vi "SetAOrange.vi"(8 "error in (no error)":errorcluster, 10 "output range":cluster{"output high":dbl, "output low":dbl}={"output high"=nan, "output low"=0.0}, 11 "MotorCtrl in":refnum<class "MotorControl.lvclass">) -> (0 "error out":errorcluster, 2 "output range dup":cluster{"output high":dbl, "output low":dbl}, 3 "MotorCtrl out":refnum<class "MotorControl.lvclass">)   [LabVIEW 2015, in "MotorControl.lvclass"]
uses:
  MotorControl.lvclass
  MotorControl.lvclass/MotorControl.ctl
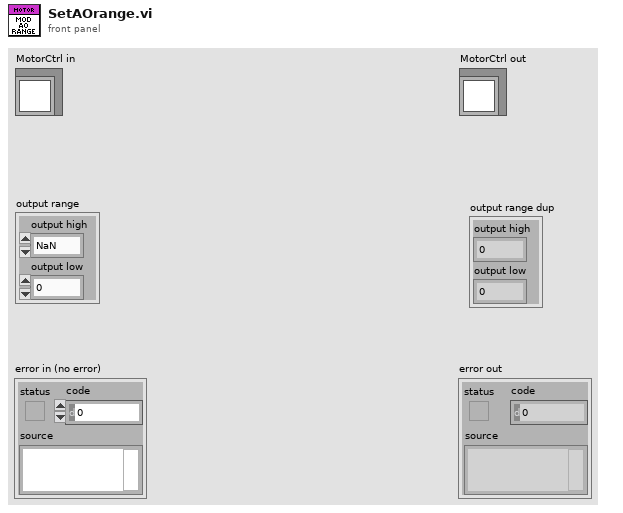
[diagram p1: front panel]
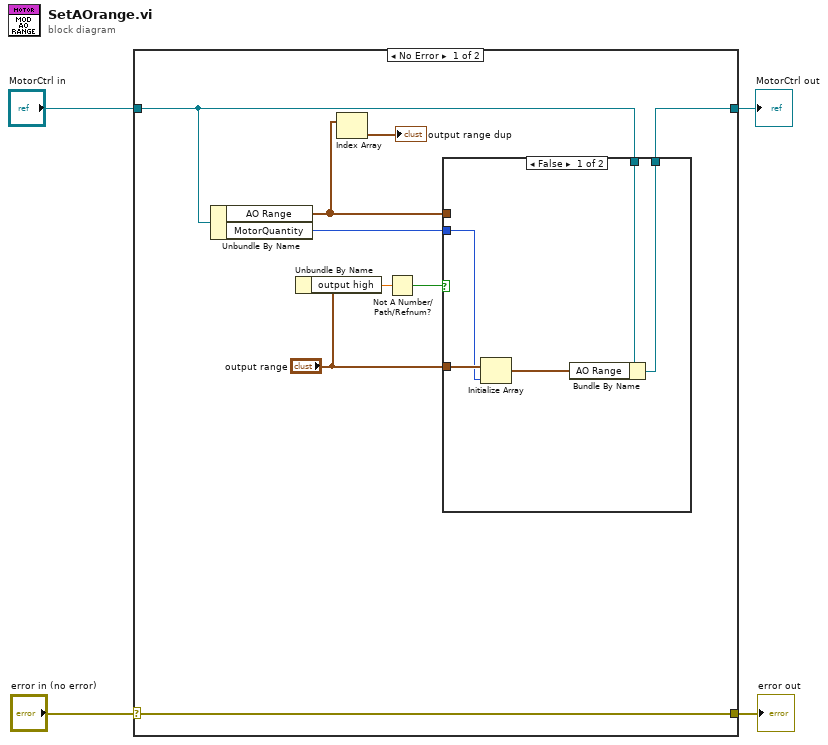
[diagram p0: block diagram]
diagram:
  n1 = case shown="No Error" "error in (no error)" {
    selector: "error in (no error)" -> [w13 w21]
    tunnel: [w13 w21] -> w3
    tunnel: [w11 w20] -> w1
    tunnel: "MotorCtrl in" -> [w12 w20]
    frame No Error {
      n2 = Unbundle By Name(w12) -> ("AO Range"=w9:cluster{"output high":dbl, "output low":dbl}[], "MotorQuantity"=w10:i32)
      n3 = Unbundle By Name("output range") -> ("output high"=w6:dbl)
      n4 = Index Array(array=w9) -> (element=→"output range dup":cluster{"output high":dbl, "output low":dbl})  [unwired: 1 in]
      n5 = Not A Number/Path/Refnum?(number/path/refnum=w6) -> (NaN/Path/Refnum?=w5:bool)
      n6 = case shown="False" w5 {
        tunnel: w12 -> [w18 w19]
        tunnel: [w17 w19] -> w11
        tunnel: w9 -> [_ _]
        tunnel: w10 -> [w14 _]
        tunnel: "output range" -> [w16 _]
        frame False {
          n7 = Initialize Array(w16, w14) -> (w15:cluster{"output high":dbl, "output low":dbl}[])
          n8 = Bundle By Name(cluster=w18, "AO Range"=w15) -> (w17:refnum<class "MotorControl.lvclass">)
        }
        frame True {
        }
      }
    }
    frame Error {
    }
  }
  "error out" <- w3
  "MotorCtrl out" <- w1
